vi "Add Worker to Worker Status Tree.vi"(4 "Worker Status":string, 7 "IP Address":string, 8 "error in (no error)":errorcluster, 9 "DC_UID":T1, 10 "WID":string, 11 "Tree Ref":refnum<vi>) -> (0 "error out":errorcluster)   [LabVIEW 2017, in "Application Manager.lvclass"]
uses:
  Application Manager.lvclass
  Common VIs/DC_UID.ctl
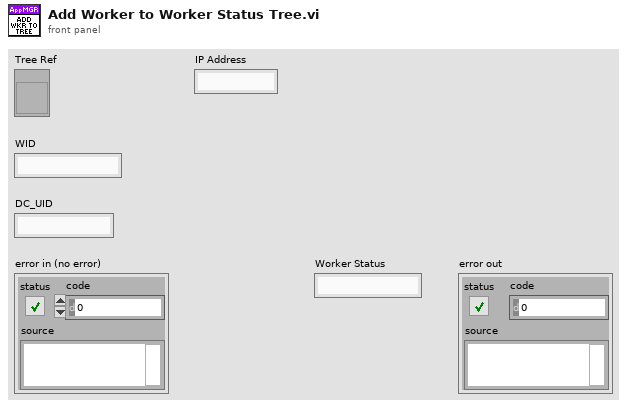
[diagram p1: front panel]
types:
  T1 = typedef "DC_UID.ctl" = string
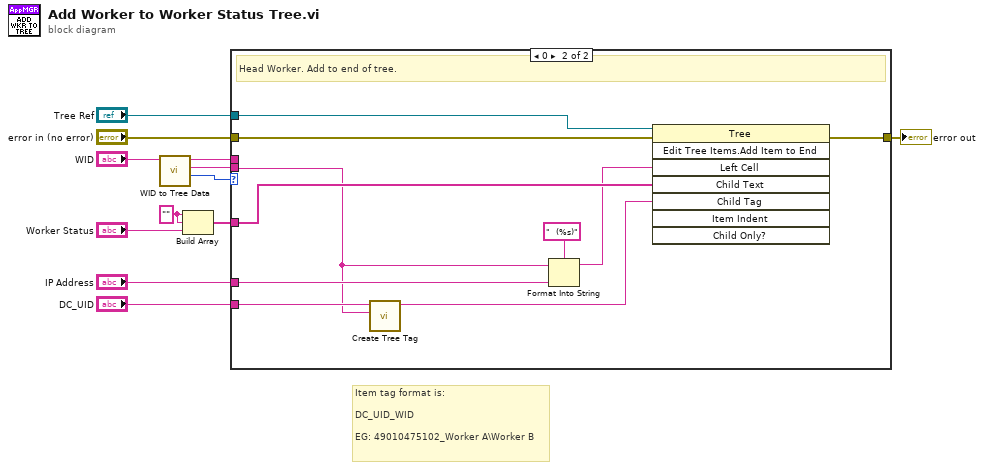
[diagram p0: block diagram]
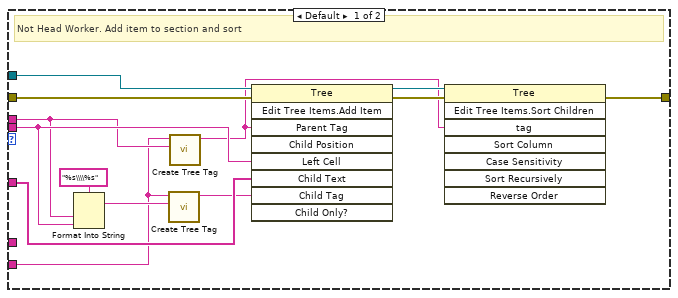
[diagram p2: hidden frame]
diagram:
  w4 = "" ("element")
  # "Item tag format is:\n\nDC_UID_WID\n\nEG: 49010475102_Worker A\\Worker B"
  n1 = call "WID to Tree Data.vi"("WID"="WID") -> ("Worker Tree Depth"=w12:i32, "Alias"=w10:string, "Owner WID"=w11:string)  [unwired: 8 in]
  n2 = Build Array(w4, w4, "Worker Status") -> (w6:string[])
  n3 = case shown="0" w12 {
    tunnel: "Tree Ref" -> [w25 w35]
    tunnel: w11 -> [w17 _]
    tunnel: w10 -> [w22 w26]
    tunnel: [w21 w34] -> w7
    tunnel: "error in (no error)" -> [w19 w29]
    tunnel: w6 -> [w18 w33]
    tunnel: "IP Address" -> [_ w30]
    tunnel: "DC_UID" -> [w14 w27]
    frame Default {
      # "Not Head Worker. Add item to section and sort"
      n4 = Format Into String(format string="%s\\\\%s", w17, w22) -> (resulting string=w15:string)  [unwired: 2 in, 1 out]
      n5 = call "Create Tree Tag.vi"("WID"=w15, "DC_UID"=w14) -> ("Tree Tag"=w13:string)  [unwired: 9 in]
      n6 = call "Create Tree Tag.vi"("WID"=w17, "DC_UID"=w14) -> ("Tree Tag"=w16:string)  [unwired: 9 in]
      n7 = invoke class="Tree" method="Edit Tree Items.Add Item"(reference=w25, error in=w19, "Parent Tag"=w16, "Left Cell"=w22, "Child Text"=w18, "Child Tag"=w13) -> (reference out=w20:refnum<vi>, error out=w24:errorcluster)  [unwired: 3 in, 7 out]
      n8 = invoke class="Tree" method="Edit Tree Items.Sort Children"(reference=w20, error in=w24, "tag"=w16) -> (error out=w21:errorcluster)  [unwired: 5 in, 7 out]
    }
    frame 0 {
      # "Head Worker. Add to end of tree."
      n9 = call "Create Tree Tag.vi"("WID"=w26, "DC_UID"=w27) -> ("Tree Tag"=w28:string)  [unwired: 9 in]
      n10 = Format Into String(format string="  (%s)", initial string=w26, w30) -> (resulting string=w31:string)  [unwired: 1 in, 1 out]
      n11 = invoke class="Tree" method="Edit Tree Items.Add Item to End"(reference=w35, error in=w29, "Left Cell"=w31, "Child Text"=w33, "Child Tag"=w28) -> (error out=w34:errorcluster)  [unwired: 3 in, 7 out]
    }
  }
  "error out" <- w7
